vi "Transfer Group.Return FIFO.Read.vi"(8 "error in (no error)":errorcluster, 9 "timeout in ms (0)":i32 format="%d ms", 11 "Transfer Group in":refnum<class "Transfer Group.lvclass">) -> (0 "error out":errorcluster, 1 "timed out?":bool, 2 "Transfer Group iteration":u64, 3 "Transfer Group out":refnum<class "Transfer Group.lvclass">)   [LabVIEW 2017, in "DSF Core.lvlib" / "Transfer Group.lvclass"]
uses:
  Transfer Group.lvclass
  Transfer Group.lvclass/Transfer Group.ctl
  Debug/Debug Flags/Debug Flags.lvclass/Debug Flags.ctl
  Debug/FIFO Flags/FIFO Flags.lvclass/FIFO Flags.ctl
  Debug/Debug Flags/Debug Flags.lvclass
  Debug/FIFO Flags/FIFO Flags.lvclass
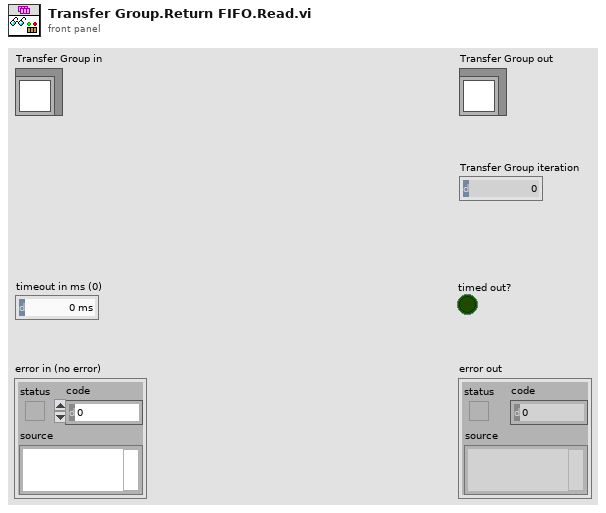
[diagram p1: front panel]
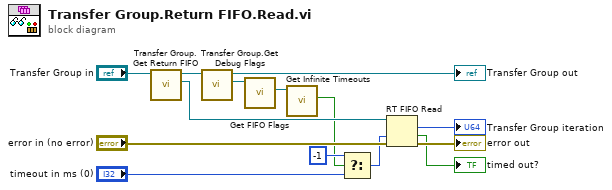
[diagram p0: block diagram]
diagram:
  n1 = call "Transfer Group.Get Return FIFO.vi"("Transfer Group in"="Transfer Group in") -> ("Return FIFO"=w13:refnum<k33>, "Transfer Group out"=w8:refnum<class "Transfer Group.lvclass">)  [unwired: 9 in]
  n2 = call "Transfer Group.Get Debug Flags.vi"("Transfer Group in"=w8) -> ("Debug Flags"=w7:refnum<class "Debug Flags.lvclass">, "Transfer Group out"=→"Transfer Group out":refnum<class "Transfer Group.lvclass">)  [unwired: 9 in]
  n3 = call "Get FIFO Flags.vi"("Debug Flags in"=w7) -> ("FIFO"=w6:refnum<class "FIFO Flags.lvclass">)  [unwired: 9 in, 1 out]
  n4 = call "Get Infinite Timeouts.vi"("FIFO Debug Flags in"=w6) -> ("infinite timeouts"=w1:bool)  [unwired: 9 in, 1 out]
  n5 = Select(t=-1, s=w1, f="timeout in ms (0)") -> (s? t:f=w3:i32)
  n6 = RT FIFO Read(0:w13, 2:w3, 3:"error in (no error)") -> (9:→"Transfer Group iteration":u64, 10:→"timed out?":bool, 11:→"error out":errorcluster)  [unwired: 1 in, 2 out]
